vi "IncrementShotFile.vi"(11 "String":string) -> ()   [LabVIEW 2013]
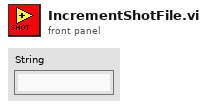
[diagram p1: front panel]
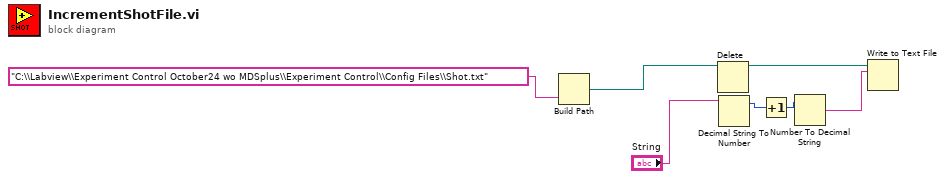
[diagram p0: block diagram]
diagram:
  n1 = Build Path(name or relative path="C:\\Labview\\Experiment Control October24 wo MDSplus\\Experiment Control\\Config Files\\Shot.txt") -> (appended path=w2:path)  [unwired: 1 in]
  n2 = Delete(path (use dialog)=w2) -> (deleted path=w4:path)  [unwired: 4 in, 2 out]
  n3 = Decimal String To Number(string="String") -> (offset past number=w5:i32)  [unwired: 2 in, 1 out]
  n4 = Increment(x=w5) -> (x+1=w6:i32)
  n5 = Number To Decimal String(number=w6) -> (decimal integer string=w7:string)  [unwired: 1 in]
  n6 = Write to Text File(file (use dialog)=w4, text=w7) -> ()  [unwired: 2 in, 3 out]
